vi "process_ref_obj.vi"(1 "input cluster":T1) -> (0 "output cluster":cluster{"destination":i16[][], dbl[]})   [LabVIEW 2010]
types:
  T1 = cluster{"Value":i32, dbl[], cluster{dbl, dbl}, "Height":u32, "Width":u32, "Image Pixels (I16)":i16[][], "Image Pixels (I16)":i16[][]}
  T2 = cluster{"Value":i32, "outy1":dbl, "outx1":dbl, "Image Pixels (I16)":i16[][]}
  T3 = cluster{"return type":i32, "return type":i32, "image":i16[][]}
  T4 = cluster{"Value":i32, "image":i16[][], "Image Pixels (I16)":i16[][], "Height":u32, "Width":u32}
  T5 = cluster{"return type":i32, "return type":i32, "destination":i16[][]}
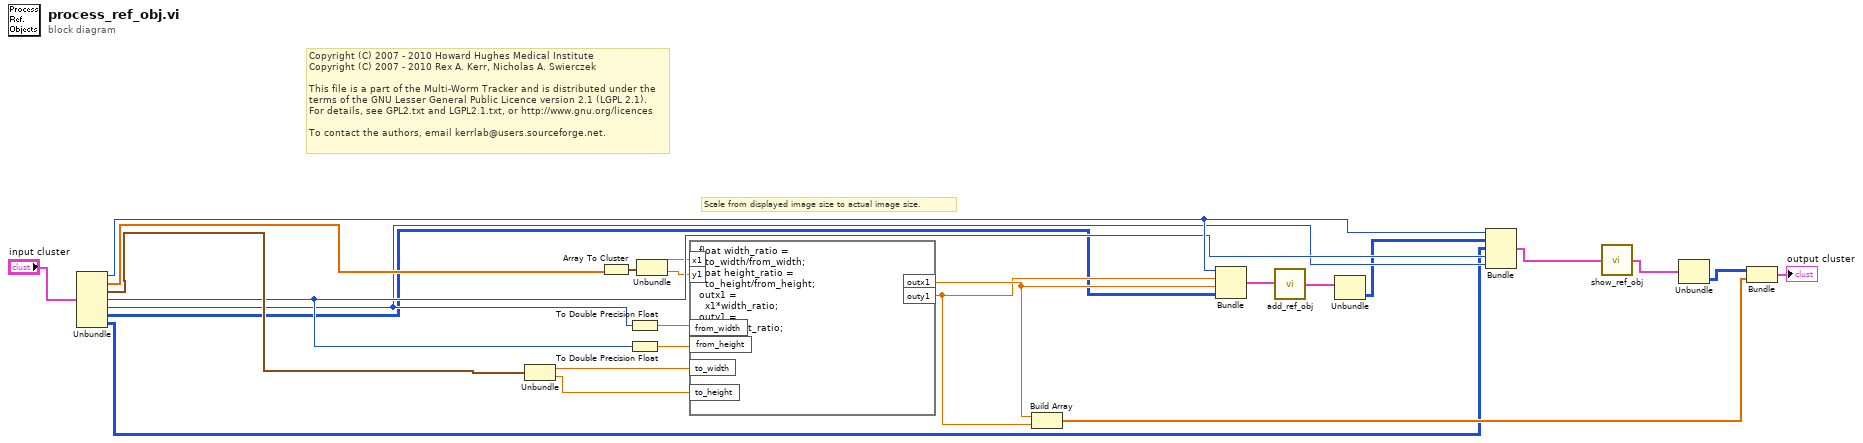
[diagram p0: block diagram]
diagram:
  # "Copyright (C) 2007 - 2010 Howard Hughes Medical Institute\nCopyright (C) 2007 - 2010 Rex A. Kerr, Nicholas A. Swierczek\n \nThis file is a part of the Multi-Worm Tracker and is distributed under the\nterms of the GNU Lesser General Public Licence version 2.1 (LGPL 2.1).\nFor details, see GPL2.txt and LGPL2.1.txt, or http://www.gnu.org/licences\n \nTo contact the authors, email kerrlab@users.sourceforge.net."
  # "Scale from displayed image size to actual image size."
  n1 = Unbundle("input cluster") -> ("Value"=w23:i32, w20:dbl[], w19:cluster{dbl, dbl}, "Height"=w18:u32, "Width"=w17:u32, "Image Pixels (I16)"=w16:i16[][], "Image Pixels (I16)"=w15:i16[][])
  n2 = Unbundle(w19) -> (w10:dbl, w9:dbl)
  n3 = Array To Cluster(array=w20) -> (cluster=w11:cluster{"[0]":dbl, "[1]":dbl})
  n4 = To Double Precision Float(number=w17) -> (double precision float=w8:dbl)
  n5 = To Double Precision Float(number=w18) -> (double precision float=w7:dbl)
  n6 = Unbundle(w11) -> ("[0]"=w6:dbl, "[1]"=w5:dbl)
  n7 = formula code="float width_ratio = \n  to_width/from_width;\nfloat height_ratio = \n  to_height/from_height;\noutx1 = \n  x1*width_ratio;\nouty1 = \n  y1*height_ratio;"("x1"=w6, "y1"=w5, "from_width"=w8, "from_height"=w7, "to_width"=w10, "to_height"=w9) -> ("outx1"=w25:dbl, "outy1"=w24:dbl)
  n8 = Build Array(w25, w24) -> (w22:dbl[])
  n9 = Bundle("Value"=w23, "outy1"=w24, "outx1"=w25, "Image Pixels (I16)"=w16) -> (w4:T2)  [unwired: 1 in]
  n10 = call "add_ref_obj.vi"("input cluster"=w4) -> ("output cluster"=w3:T3)
  n11 = Unbundle(w3) -> ("image"=w14:i16[][])  [unwired: 2 out]
  n12 = Bundle("Value"=w23, "image"=w14, "Image Pixels (I16)"=w15, "Height"=w18, "Width"=w17) -> (w2:T4)  [unwired: 1 in]
  n13 = call "show_ref_obj.vi"("input cluster"=w2) -> ("output cluster"=w1:T5)
  n14 = Unbundle(w1) -> ("destination"=w13:i16[][])  [unwired: 2 out]
  n15 = Bundle("destination"=w13, w22) -> (→"output cluster":cluster{"destination":i16[][], dbl[]})  [unwired: 1 in]
